vi "Jobs - Config File.vi"(6 "Action":enum16{"Write", "Read", "Read All", "Remove"}(ring)=enum."Read", 7 "Remove Section?":bool=TRUE, 8 "error in (no error)":errorcluster, 9 "Value":string[](array[string]), 10 "Key Name":string[](array[string]), 11 "Jobs No":string) -> (0 "error out":errorcluster, 2 "key names":string[](array[string]), 3 "Value Out":T1(array[cluster]))   [LabVIEW 2019]
uses:
  <vilib>/Utility/config.llb/Write Key (String).vi
  <vilib>/Utility/config.llb/Read Key (String).vi
  <vilib>/Utility/config.llb/NI_LVConfig.lvlib
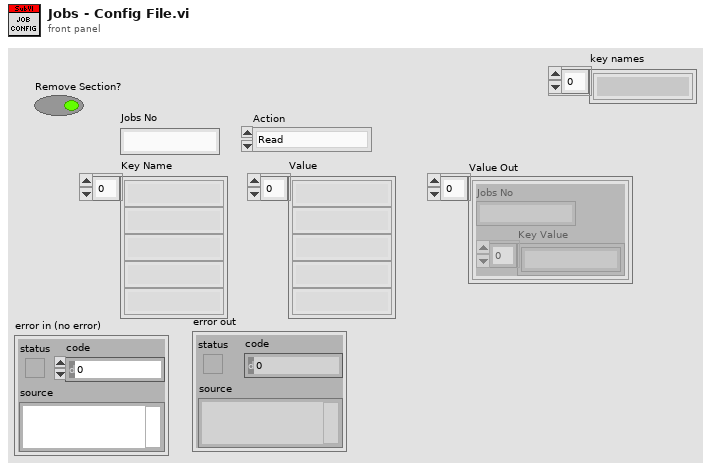
[diagram p1: front panel]
types:
  T1 = cluster{"Jobs No":string, "Key Value":string[]}[]
  T2 = typedef "NI_LVConfig.lvlib/Config Data RefNum.ctl" = refnum<k1>
  T3 = cluster{"Station Name":string, "Key Value":string[]}
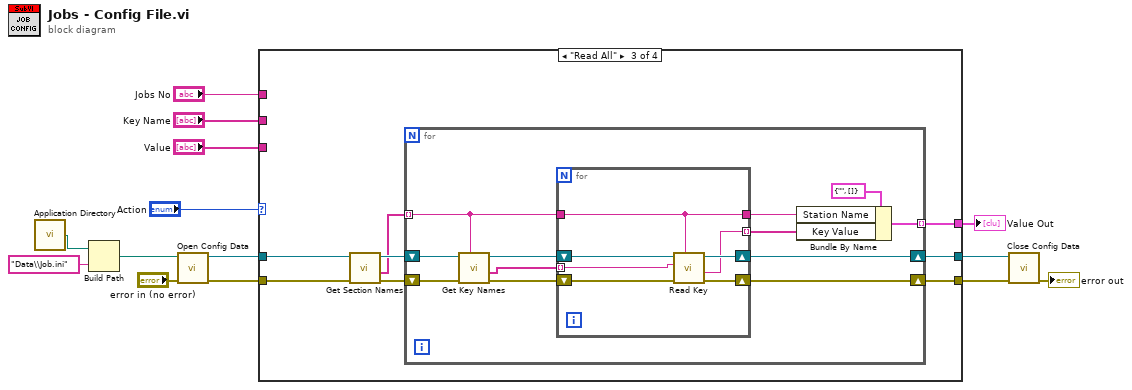
[diagram p0: block diagram]
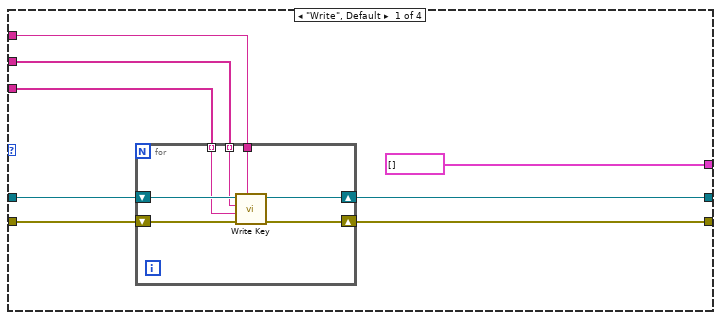
[diagram p2: hidden frame]
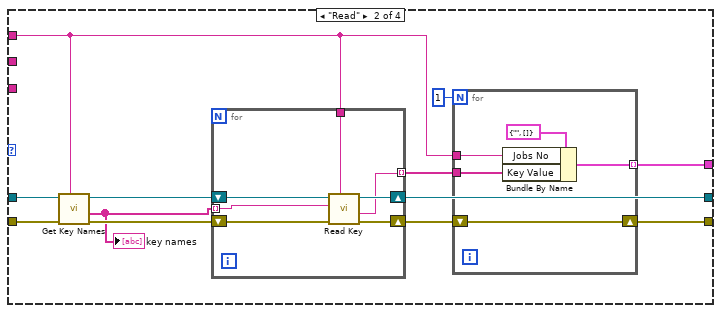
[diagram p3: hidden frame]
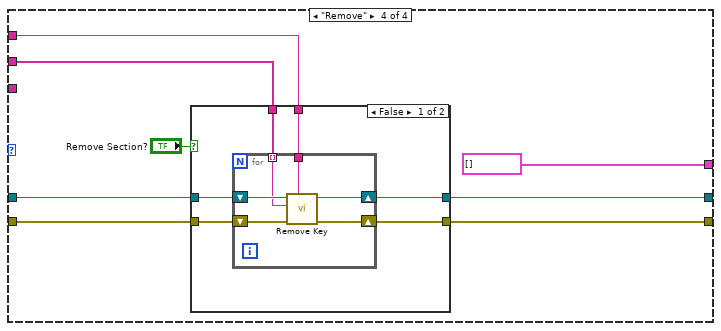
[diagram p4: hidden frame]
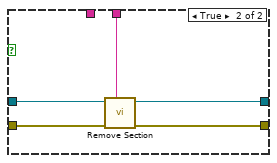
[diagram p5: hidden frame]
diagram:
  n1 = call <vilib>:"Application Directory.vi"() -> ("Application Directory"=w14:path)
  n2 = Build Path(base path=w14, name or relative path="Data\\Job.ini") -> (appended path=w1:path)
  n3 = call <vilib>:"Open Config Data.vi"("error in (no error)"="error in (no error)", "configuration file path"=w1) -> ("error out"=w12:errorcluster, "refnum"=w11:T2)  [unwired: 7 in, 1 out]
  n4 = case shown="\"Read All\"" "Action" {
    tunnel: w12 -> [w22 w33 w58 w86]
    tunnel: w11 -> [w21 w34 w57 w88]
    tunnel: [w20 w41 w60 w87] -> w10
    tunnel: [w19 w37 w61 w85] -> w9
    tunnel: "Value" -> [w18 _ _ _]
    tunnel: "Key Name" -> [w17 _ _ w81]
    tunnel: "Jobs No" -> [w16 w31 _ w84]
    tunnel: [cluster{"Station Name":string, "Key":string[]}[] [] w39 w59 cluster{"Station Name":string, "Key":string[]}[] []] -> w2
    frame "Write", Default {
      n5 = for {
        shift-right: [w26] -> w19
        shift-left: w22 -> [w29]
        shift-right: [w27] -> w20
        shift-left: w21 -> [w28]
        tunnel: w16 -> [w25]
        tunnel: w17 -> [w24] mode=indexing
        tunnel: w18 -> [w23] mode=indexing
        n6 = call-poly <vilib>:"Write Key.vi"("section"=w25, "error in (no error)"=w29, "value"=w23, "key"=w24, "refnum"=w28) -> ("error out"=w26:errorcluster, "refnum out"=w27:T2)  [unwired: 4 in, 1 out]
      }
    }
    frame "Read" {
      n7 = call <vilib>:"Get Key Names.vi"("section"=w31, "error in (no error)"=w33, "refnum"=w34) -> ("error out"=w32:errorcluster, "key names"=w30:string[], "refnum out"=w35:T2)  [unwired: 5 in, 1 out]
      "key names" <- w30
      n8 = for {
        tunnel: w31 -> [w49]
        shift-right: [w50] -> w41
        shift-left: w35 -> [w53]
        shift-right: [w51] -> w36
        shift-left: w32 -> [w52]
        tunnel: [w48] -> w40 mode=indexing
        tunnel: w30 -> [w47] mode=indexing
        n9 = call-poly <vilib>:"Read Key.vi"("section"=w49, "error in (no error)"=w52, "key"=w47, "refnum"=w53) -> ("error out"=w51:errorcluster, "value"=w48:string, "refnum out"=w50:T2)  [unwired: 4 in, 1 out]
      }
      n10 = for {
        N: 1 -> [_]
        tunnel: w31 -> [w45]
        tunnel: w40 -> [w44]
        tunnel: [w43] -> w39 mode=indexing
        shift-right: [w42] -> w37
        shift-left: w36 -> [w42]
        n11 = Bundle By Name(cluster=cluster{"Jobs No":string, "Key Value":string[]} {"Jobs No"="", "Key Value"=[]}, "Jobs No"=w45, "Key Value"=w44) -> (w43:cluster{"Jobs No":string, "Key Value":string[]})
      }
    }
    frame "Read All" {
      n12 = call <vilib>:"Get Section Names.vi"("error in (no error)"=w58, "refnum"=w57) -> ("error out"=w56:errorcluster, "section names"=w54:string[], "refnum out"=w55:T2)  [unwired: 7 in]
      n13 = for {
        tunnel: [w62] -> w59 mode=indexing
        shift-right: [w73] -> w61
        shift-left: w56 -> [w71]
        shift-right: [w72] -> w60
        shift-left: w55 -> [w69]
        tunnel: w54 -> [w66] mode=indexing
        n14 = call <vilib>:"Get Key Names.vi"("section"=w66, "error in (no error)"=w71, "refnum"=w69) -> ("error out"=w70:errorcluster, "key names"=w67:string[], "refnum out"=w68:T2)  [unwired: 5 in, 1 out]
        n15 = for {
          shift-right: [w77] -> w72
          shift-left: w68 -> [w80]
          shift-right: [w78] -> w73
          shift-left: w70 -> [w79]
          tunnel: [w76] -> w63 mode=indexing
          tunnel: w67 -> [w75] mode=indexing
          tunnel: w66 -> [w74]
          tunnel: [w74] -> w64
          n16 = call-poly <vilib>:"Read Key.vi"("section"=w74, "error in (no error)"=w79, "key"=w75, "refnum"=w80) -> ("error out"=w78:errorcluster, "value"=w76:string, "refnum out"=w77:T2)  [unwired: 4 in, 1 out]
        }
        n17 = Bundle By Name(cluster=T3 {"Station Name"="", "Key Value"=[]}, "Station Name"=w64, "Key Value"=w63) -> (w62:T3)
      }
    }
    frame "Remove" {
      n18 = case shown="False" "Remove Section?" {
        tunnel: w88 -> [w94 w105]
        tunnel: [w91 w104] -> w87
        tunnel: w86 -> [w93 w103]
        tunnel: [w92 w102] -> w85
        tunnel: w84 -> [w90 w101]
        tunnel: w81 -> [w89 _]
        frame False {
          n19 = for {
            tunnel: w90 -> [w96]
            shift-right: [w97] -> w91
            shift-left: w94 -> [w100]
            shift-right: [w98] -> w92
            shift-left: w93 -> [w99]
            tunnel: w89 -> [w95] mode=indexing
            n20 = call <vilib>:"Remove Key.vi"("section"=w96, "error in (no error)"=w99, "key"=w95, "refnum"=w100) -> ("error out"=w98:errorcluster, "refnum out"=w97:T2)  [unwired: 5 in, 1 out]
          }
        }
        frame True {
          n21 = call <vilib>:"Remove Section.vi"("section"=w101, "error in (no error)"=w103, "refnum"=w105) -> ("error out"=w102:errorcluster, "refnum out"=w104:T2)  [unwired: 6 in, 1 out]
        }
      }
    }
  }
  "Value Out" <- w2
  n22 = call <vilib>:"Close Config Data.vi"("error in (no error)"=w9, "refnum"=w10) -> ("error out"=→"error out":errorcluster)  [unwired: 8 in, 1 out]
